vi "xeva-getImage.vi"(3 "error in (no error)":errorcluster, 4 "xeva-dimensions":cluster{"Width":u32, "Height":u32}={"Width"=320, "Height"=256}, 5 "xeva-camref":T1=refnum) -> (0 "error out":errorcluster, 1 "xeva-histogram":T2(graph)={"X Values"=[381.555, 1026.665, 1671.775, 2316.885, 2961.995, 3607.105, 4252.215, 4897.325, 5542.435, 6187.545, 6832.655, 7477.765, 8122.875, 8767.985, 9413.095, 10058.205, 10703.315, 11348.425, 11993.535, 12638.645, 13283.755, 13928.865, 14573.975, 15219.085, 15864.195, 16509.305, 17154.415, 17799.525, 18444.635, 19089.745, 19734.855, 20379.965, 21025.075, 21670.185, 22315.295, 22960.405, 23605.515, 24250.625, 24895.735, 25540.845, 26185.955, 26831.065, 27476.175, 28121.285, 28766.395, 29411.505, 30056.615, 30701.725, 31346.835, 31991.945, 32637.055, 33282.165, 33927.275, 34572.385, 35217.495, 35862.605, 36507.715, 37152.825, 37797.935, 38443.045, 39088.155, 39733.265, 40378.375, 41023.485, 41668.595, 42313.705, 42958.815, 43603.925, 44249.035, 44894.145, 45539.255, 46184.365, 46829.475, 47474.585, 48119.695, 48764.805, 49409.915, 50055.025, 50700.135, 51345.245, 51990.355, 52635.465, 53280.575, 53925.685, 54570.795, 55215.905, 55861.015, 56506.125, 57151.235, 57796.345, 58441.455, 59086.565, 59731.675, 60376.785, 61021.895, 61667.005, 62312.115, 62957.225, 63602.335, 64247.445], "Histogram: h(x)"=[235, 173, 0, 115, 75, 0, 36, 38, 0, 21, 0, 14, 13, 0, 16, 28, 0, 49, 0, 91, 118, 0, 184, 328, 0, 436, 626, 0, 854, 0, 1158, 1443, 0, 1891, 2217, 0, 2808, 0, 3354, 3711, 0, 4252, 4588, 0, 4786, 0, 4898, 4792, 0, 4596, 4273, 0, 3970, 3545, 0, 3221, 0, 3015, 2668, 0, 2533, 2324, 0, 2214, 0, 2124, 1991, 0, 1897, 1839, 0, 1906, 0, 1861, 1832, 0, 1883, 1841, 0, 1844, 1875, 0, 1813, 0, 1765, 1729, 0, 1611, 1524, 0, 1290, 0, 1154, 968, 0, 749, 585, 0, 491, 313]}, 2 "xeva-data":u16[][](array[numeric]))   [LabVIEW 2015]
doc: "This example shows how to open the camera, grab frames and display them on the control-panel. To get a better visualisation the histogram is spread."
uses:
  <vilib>/Xenics Infrared Solutions/Xeneth LabVIEW API/VIs/Controls/Camara.ctl
  <vilib>/Xenics Infrared Solutions/Xeneth LabVIEW API/VIs/Controls/FrameType.ctl
  <vilib>/picture/picture.llb/Draw 8-Bit Pixmap.vi
  <vilib>/Analysis/NI_AALBase.lvlib
  <vilib>/Xenics Infrared Solutions/Xeneth LabVIEW API/Xeneth.lvlib
panel:
  out "cam":picture
  # "This example shows how to open the camera, grab frames and display them on the control-panel. \nTo get a better visualisation the histogram is spread. The picture can although be acquired using GetPicture.vi. \nThe code inside the while-loop essentially the same. Here a 16 Bit Camera is assumed."
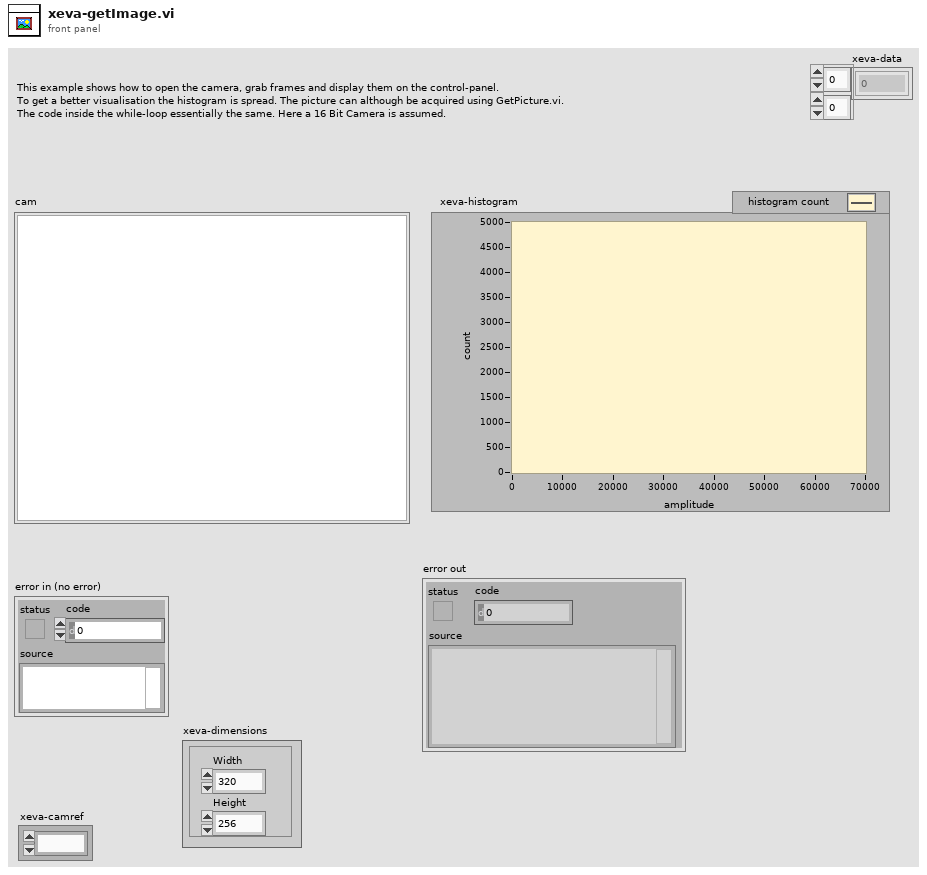
[diagram p1: front panel]
types:
  T1 = typedef "Xeneth.lvlib/Camara.ctl" = refnum<k1>
  T2 = cluster{"X Values":dbl[], "Histogram: h(x)":i32[]}
  T3 = typedef "Xeneth.lvlib/FrameType.ctl" = u32
  T4 = enum16{"big-endian, network order", "native, host order", "little-endian"}
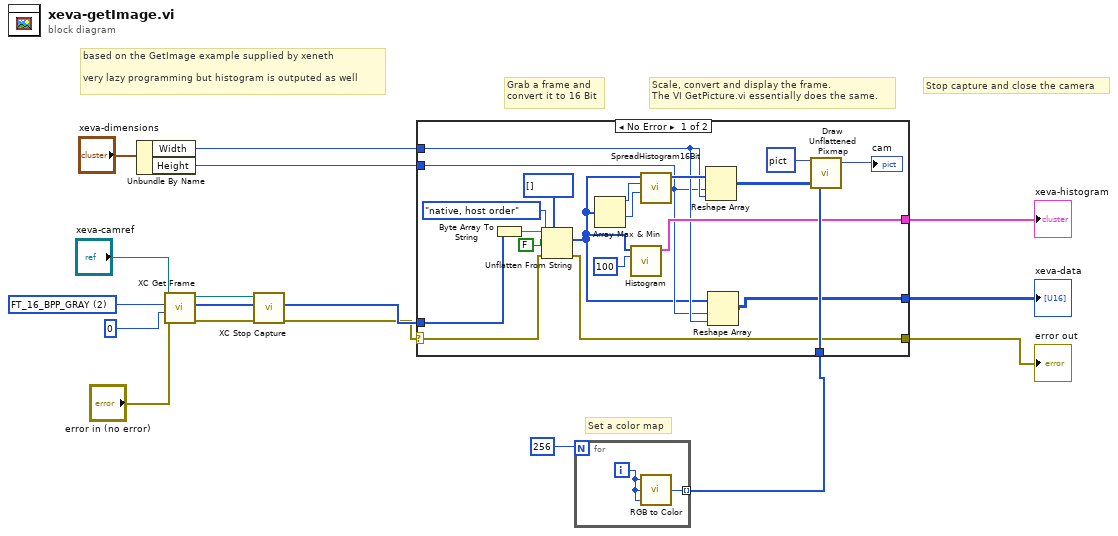
[diagram p0: block diagram]
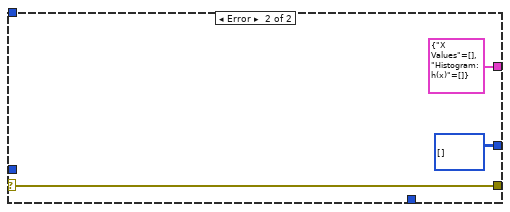
[diagram p2: hidden frame]
diagram:
  w13 = T3 2 items=["FT_NATIVE", "FT_8_BPP_GRAY", "FT_16_BPP_GRAY", "FT_32_BPP_GRAY", "FT_32_BPP_RGBA", "FT_32_BPP_RGB", "FT_32_BPP_BGRA", "FT_32_BPP_BGR"] ("type")
  # "based on the GetImage example supplied by xeneth\n\nvery lazy programming but histogram is outputed as well"
  # "Grab a frame and \nconvert it to 16 Bit"
  # "Scale, convert and display the frame.\nThe VI GetPicture.vi essentially does the same."
  # "Stop capture and close the camera"
  # "Set a color map"
  n1 = Unbundle By Name("xeva-dimensions") -> ("Width"=w3:u32, "Height"=w2:u32)
  n2 = call <vilib>:"XC Get Frame.vi"("error in (no error)"="error in (no error)", "uFlags"=0, "type"=w13, "Cam Ref 2"="xeva-camref") -> ("error out"=w7:errorcluster, "buffer"=w12:u8[], "Cam Ref Out"=w14:T1)  [unwired: 5 in]
  n3 = call <vilib>:"XC Stop Capture.vi"("error in (no error)"=w7, "Cam Ref"=w14) -> ("error out"=w6:errorcluster)  [unwired: 8 in, 1 out]
  n4 = for {
    N: 256 -> [_]
    tunnel: [w18] -> w15 mode=indexing
    i -> [w17]
    n5 = call <vilib>:"RGB to Color.vi"("B"=w17, "G"=w17, "R"=w17) -> ("Color"=w18:u32)
  }
  n6 = case shown="No Error" w6 {
    selector: w6 -> [w24 w39]
    tunnel: w15 -> [w37 _]
    tunnel: w2 -> [w21 _]
    tunnel: w3 -> [w22 _]
    tunnel: w12 -> [w29 _]
    tunnel: [w28 w39] -> w1
    tunnel: [w23 T2 {"X Values"=[], "Histogram: h(x)"=[]} ("Histogram Graph")] -> w10
    tunnel: [w19 u16[][] [] ("Data")] -> w8
    frame No Error {
      n7 = Byte Array To String(unsigned byte array=w29) -> (string=w33:string)
      n8 = Unflatten From String(type=u16[] [] ("Data"), binary string=w33, data includes array or string size? (T)=FALSE, byte order (0:big-endian, network order)=T4."native, host order", error in (no error)=w24) -> (value=w20:u16[], error out=w28:errorcluster)  [unwired: 1 out]
      n9 = Array Max & Min(array=w20) -> (max value=w25:u16, min value=w26:u16)  [unwired: 2 out]
      n10 = call <vilib>:"Histogram.vi"("intervals"=100, "X"=w20) -> ("Histogram Graph"=w23:T2)  [unwired: 6 in, 3 out]
      n11 = call <vilib>:"SpreadHistogram16Bit.vi"("min"=w26, "max"=w25, "buffer"=w20) -> ("Array"=w27:u8[])  [unwired: 8 in]
      n12 = Reshape Array(w27, w21, w22) -> (w35:u8[][])
      n13 = Reshape Array(w20, w21, w22) -> (w19:u16[][])
      n14 = call-poly <vilib>:"Draw Unflattened Pixmap.vi"("picture"=picture data[5B], "data"=w35, "color table"=w37) -> ("new picture"=→"cam":picture)  [unwired: 6 in]
    }
    frame Error {
    }
  }
  "error out" <- w1
  "xeva-histogram" <- w10
  "xeva-data" <- w8
